vi "array - sorted inexes.vi"(11 "x":dbl[](array[numeric])=[1.0, 5.0, 3.0, 7.0, 0.0]) -> (1 "index array":i32[](array[numeric]), 2 "sorted array":dbl[](array[numeric]))   [LabVIEW 2020]
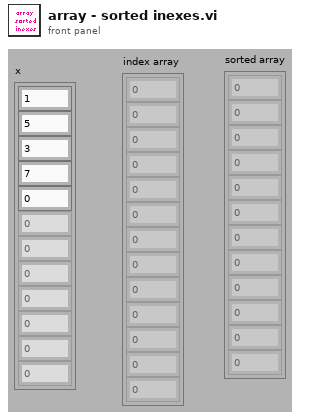
[diagram p1: front panel]
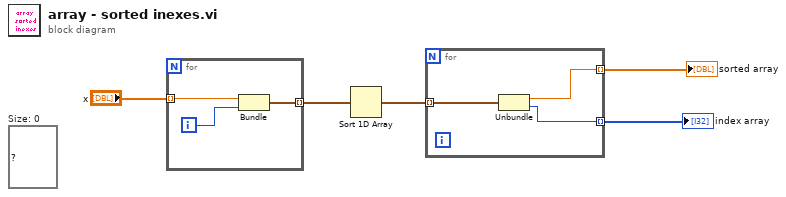
[diagram p0: block diagram]
diagram:
  (unwired) map{i32, dbl} {}  # Size: 0
  n1 = for {
    tunnel: "x" -> [w7] mode=indexing
    tunnel: [w8] -> w4 mode=indexing
    i -> [w6]
    n2 = Bundle(w7, w6) -> (w8:cluster{dbl, i32})  [unwired: 1 in]
  }
  n3 = Sort 1D Array(array=w4) -> (sorted array=w3:cluster{dbl, i32}[])
  n4 = for {
    tunnel: w3 -> [w11] mode=indexing
    tunnel: [w10] -> w2 mode=indexing
    tunnel: [w9] -> w1 mode=indexing
    n5 = Unbundle(w11) -> (w9:dbl, w10:i32)
  }
  "index array" <- w2
  "sorted array" <- w1
